vi "CMD_SET_PARAMS.vi"(8 "Max Vel":i32=99, 9 "Chan Ident":string="1", 10 "Accel":i32) -> (0 "ReqCmd":string, 1 "ParamsCmd":string)   [LabVIEW 2017]
panel:
  out "连接的字符串":string
  out "MinVelocity":string
  out "MaxVel":string
  out "Accel":string
  # "（Max Speed/mm）"
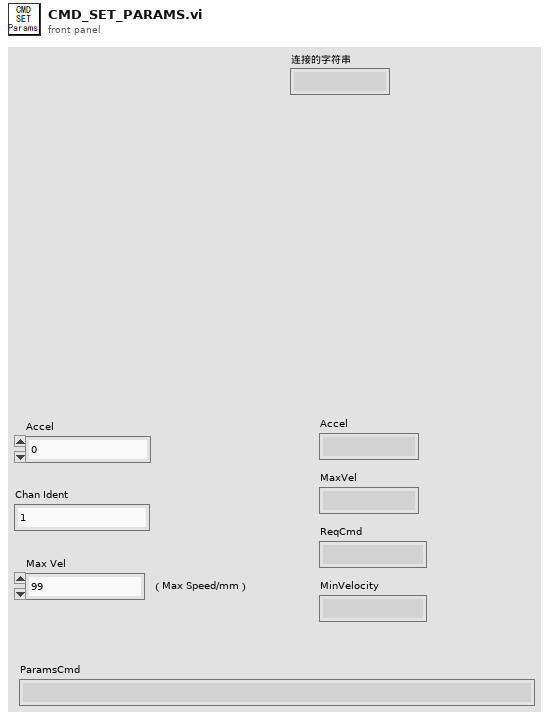
[diagram p1: front panel]
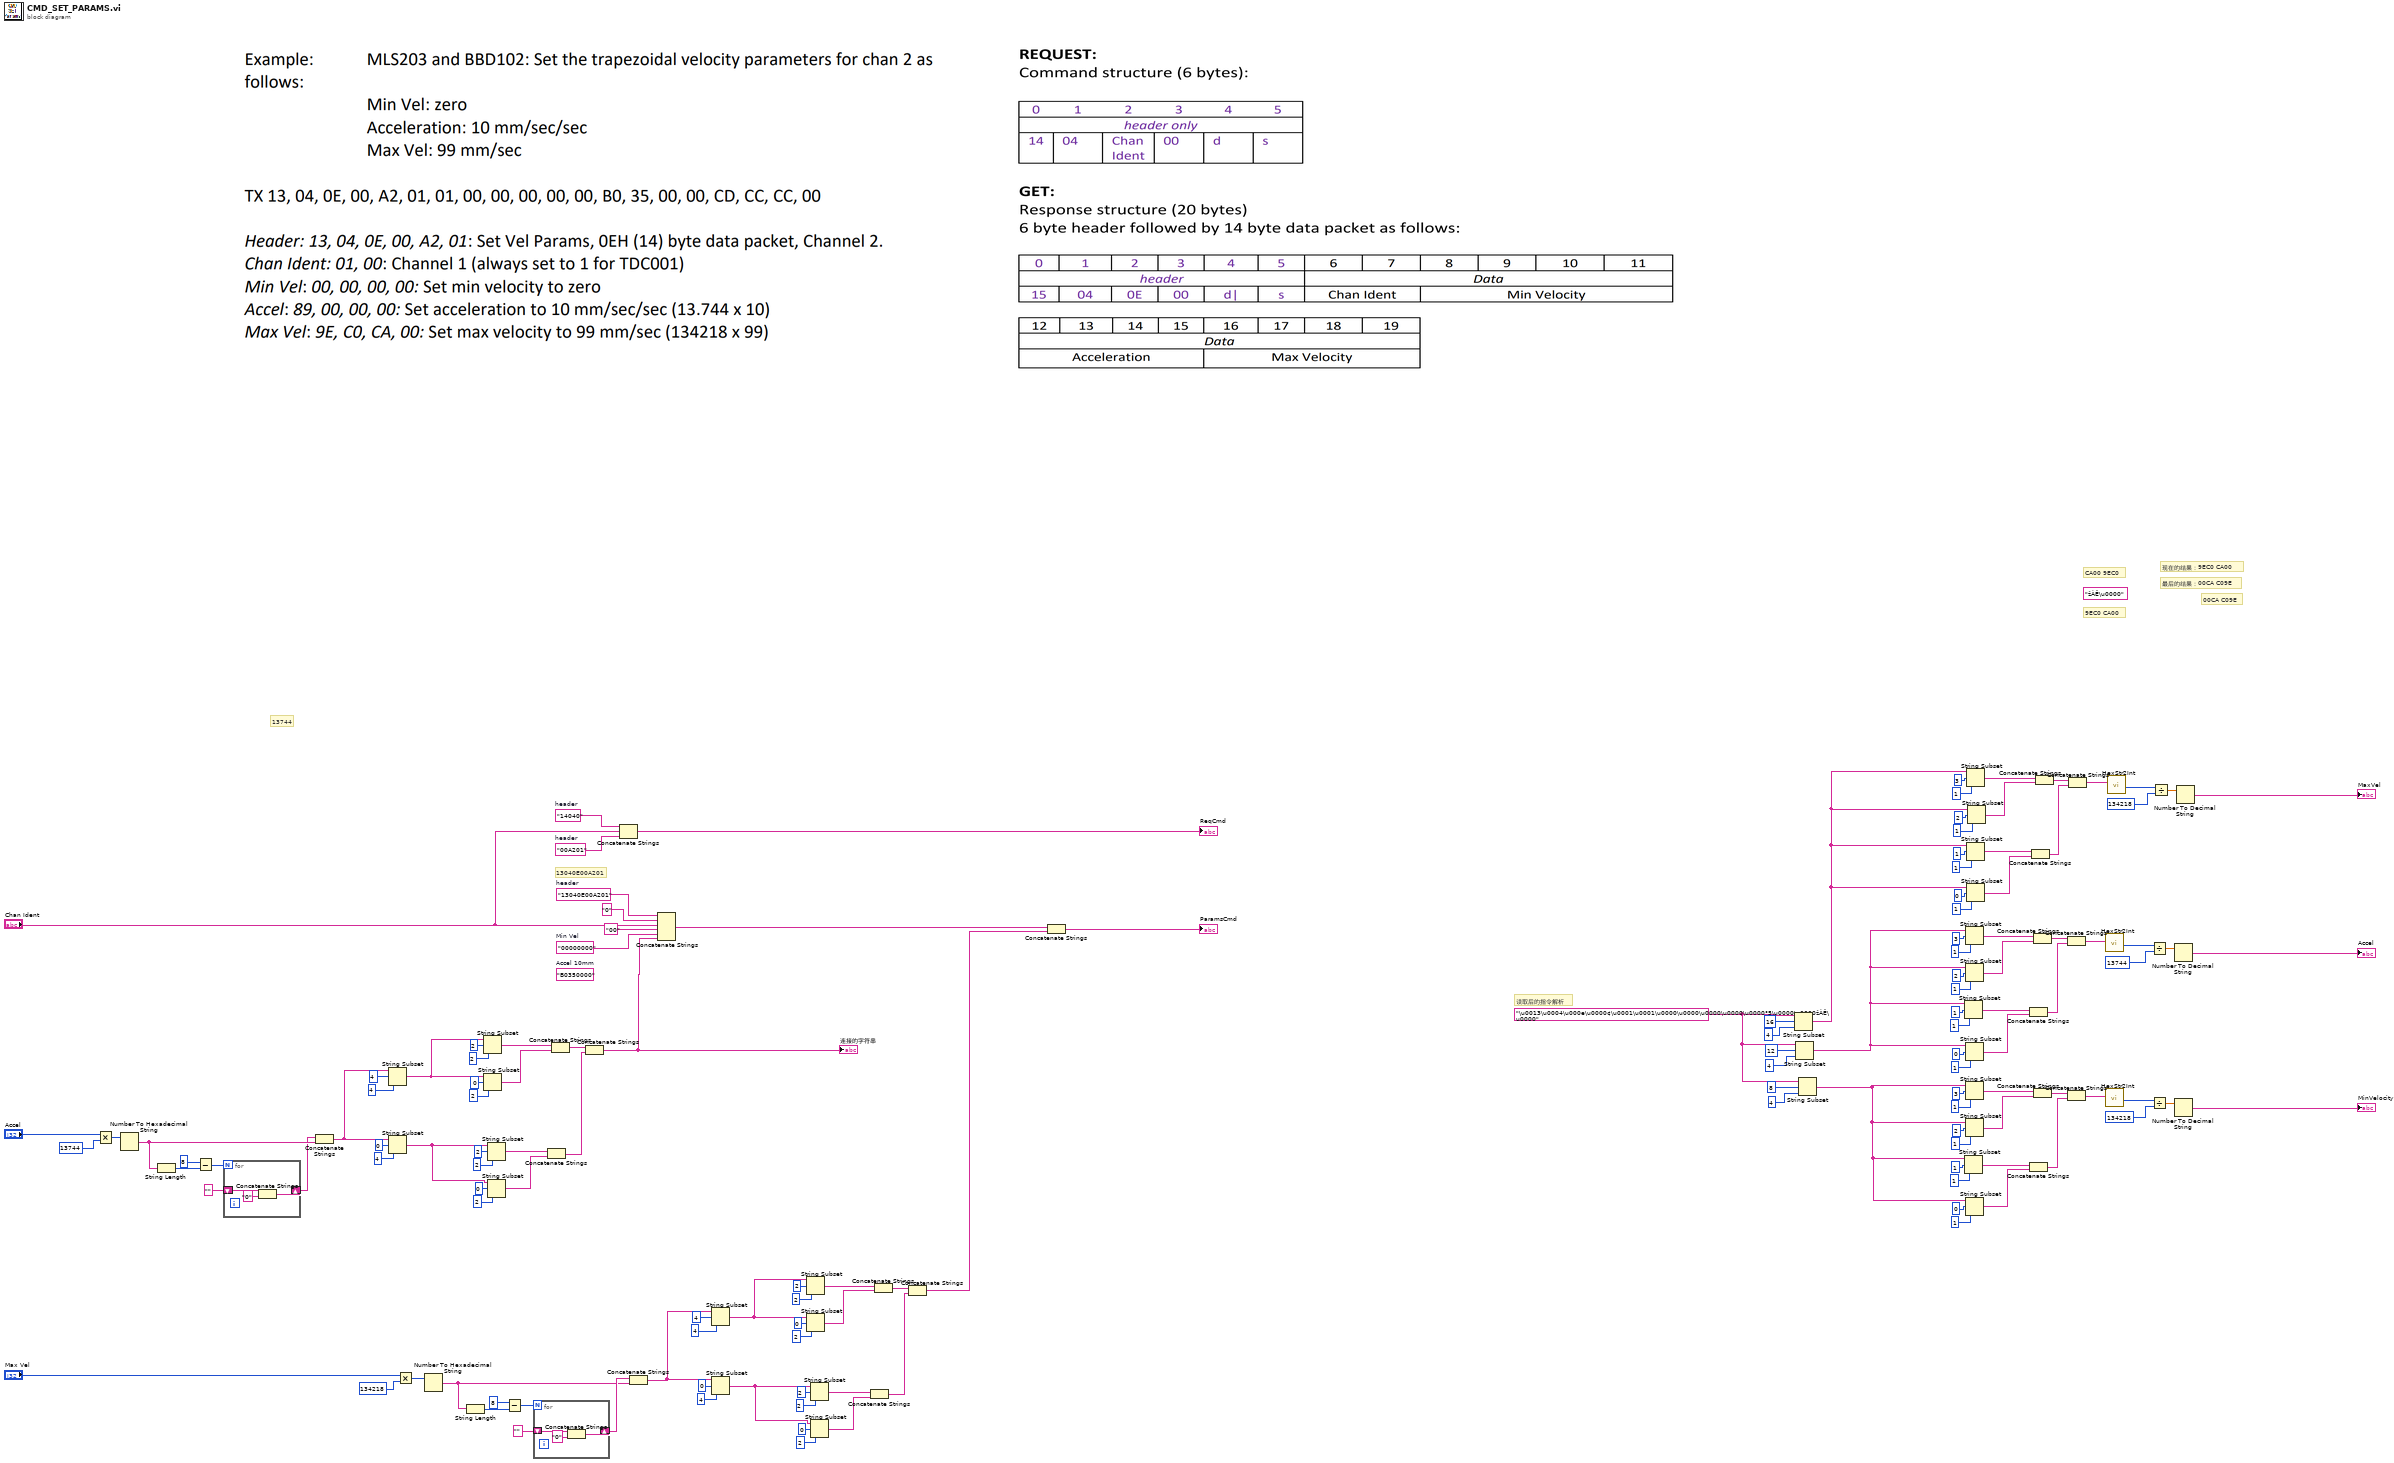
[diagram p0: block diagram]
diagram:
  (unwired) "žÀÊ\u0000" ("MaxVelocity 2")
  w92 = "\u0013\u0004\u000e\u0000¢\u0001\u0001\u0000\u0000\u0000\u0000\u0000°5\u0000\u0000žÀÊ\u0000" ("Hex Display")
  w101 = "00A201"  # header
  w103 = "14040"  # header
  (unwired) "B0350000"  # Accel 10mm
  w108 = "00000000"  # Min Vel
  w110 = "13040E00A201"  # header
  # "13744"
  # "00CA C09E"
  # "现在的结果：9EC0 CA00"
  # "9EC0 CA00"
  # "CA00 9EC0"
  # "最后的结果：00CA C09E"
  # "读取后的指令解析"
  # "13040E00A201"
  n1 = Multiply(x="Accel", y=13744) -> (x*y=w30:i32)
  n2 = Number To Hexadecimal String(2:w30) -> (0:w31:string)  [unwired: 1 in]
  n3 = String Length(string=w31) -> (length=w4:i32)
  n4 = Subtract(x=8, y=w4) -> (x-y=w5:i32)
  n5 = for {
    N: w5 -> [_]
    shift-right: [w140] -> w7
    shift-left: "" -> [w142]
    n6 = Concatenate Strings(w142, "0" ("字符串")) -> (w140:string)
  }
  n7 = Concatenate Strings(w7, w31) -> (w12:string)
  n8 = String Subset(string=w12, offset (0)=4 ("偏移量(0)"), length (rest)=4 ("长度（剩余）")) -> (substring=w17:string)
  n9 = String Subset(string=w12, offset (0)=0 ("偏移量(0)"), length (rest)=4 ("长度（剩余）")) -> (substring=w24:string)
  n10 = Multiply(x="Max Vel", y=134218) -> (x*y=w105:i32)
  n11 = Number To Hexadecimal String(2:w105) -> (0:w104:string)  [unwired: 1 in]
  n12 = String Length(string=w104) -> (length=w138:i32)
  n13 = String Subset(string=w17, offset (0)=2 ("偏移量(0)"), length (rest)=2 ("长度（剩余）")) -> (substring=w18:string)
  n14 = String Subset(string=w17, offset (0)=0 ("偏移量(0)"), length (rest)=2 ("长度（剩余）")) -> (substring=w19:string)
  n15 = String Subset(string=w24, offset (0)=2 ("偏移量(0)"), length (rest)=2 ("长度（剩余）")) -> (substring=w25:string)
  n16 = String Subset(string=w24, offset (0)=0 ("偏移量(0)"), length (rest)=2 ("长度（剩余）")) -> (substring=w26:string)
  n17 = Subtract(x=8, y=w138) -> (x-y=w137:i32)
  n18 = for {
    N: w137 -> [_]
    shift-right: [w143] -> w135
    shift-left: "" -> [w145]
    n19 = Concatenate Strings(w145, "0" ("字符串")) -> (w143:string)
  }
  n20 = Concatenate Strings(w25, w26) -> (w28:string)
  n21 = Concatenate Strings(w18, w19) -> (w27:string)
  n22 = Concatenate Strings(w27, w28) -> (w1:string)
  "连接的字符串" <- w1
  n23 = Concatenate Strings(w103, "Chan Ident", w101) -> (→"ReqCmd":string)
  n24 = Concatenate Strings(w135, w104) -> (w130:string)
  n25 = Concatenate Strings(w110, "0" ("字符串"), "Chan Ident", "00" ("字符串"), w108, w1) -> (w109:string)
  n26 = String Subset(string=w130, offset (0)=4 ("偏移量(0)"), length (rest)=4 ("长度（剩余）")) -> (substring=w125:string)
  n27 = String Subset(string=w130, offset (0)=0 ("偏移量(0)"), length (rest)=4 ("长度（剩余）")) -> (substring=w118:string)
  n28 = String Subset(string=w125, offset (0)=2 ("偏移量(0)"), length (rest)=2 ("长度（剩余）")) -> (substring=w124:string)
  n29 = String Subset(string=w125, offset (0)=0 ("偏移量(0)"), length (rest)=2 ("长度（剩余）")) -> (substring=w123:string)
  n30 = String Subset(string=w118, offset (0)=2 ("偏移量(0)"), length (rest)=2 ("长度（剩余）")) -> (substring=w117:string)
  n31 = String Subset(string=w118, offset (0)=0 ("偏移量(0)"), length (rest)=2 ("长度（剩余）")) -> (substring=w116:string)
  n32 = Concatenate Strings(w117, w116) -> (w114:string)
  n33 = Concatenate Strings(w124, w123) -> (w115:string)
  n34 = Concatenate Strings(w115, w114) -> (w113:string)
  n35 = Concatenate Strings(w109, w113) -> (→"ParamsCmd":string)
  n36 = String Subset(string=w92, offset (0)=16 ("偏移量(0)"), length (rest)=4 ("长度（剩余）")) -> (substring=w74:string)
  n37 = String Subset(string=w92, offset (0)=12 ("偏移量(0)"), length (rest)=4 ("长度（剩余）")) -> (substring=w53:string)
  n38 = String Subset(string=w92, offset (0)=8 ("偏移量(0)"), length (rest)=4 ("长度（剩余）")) -> (substring=w32:string)
  n39 = String Subset(string=w53, offset (0)=1 ("偏移量(0)"), length (rest)=1 ("长度（剩余）")) -> (substring=w64:string)
  n40 = String Subset(string=w32, offset (0)=1 ("偏移量(0)"), length (rest)=1 ("长度（剩余）")) -> (substring=w43:string)
  n41 = String Subset(string=w53, offset (0)=3 ("偏移量(0)"), length (rest)=1 ("长度（剩余）")) -> (substring=w58:string)
  n42 = String Subset(string=w53, offset (0)=0 ("偏移量(0)"), length (rest)=1 ("长度（剩余）")) -> (substring=w65:string)
  n43 = String Subset(string=w32, offset (0)=3 ("偏移量(0)"), length (rest)=1 ("长度（剩余）")) -> (substring=w37:string)
  n44 = String Subset(string=w32, offset (0)=0 ("偏移量(0)"), length (rest)=1 ("长度（剩余）")) -> (substring=w44:string)
  n45 = String Subset(string=w53, offset (0)=2 ("偏移量(0)"), length (rest)=1 ("长度（剩余）")) -> (substring=w59:string)
  n46 = String Subset(string=w32, offset (0)=2 ("偏移量(0)"), length (rest)=1 ("长度（剩余）")) -> (substring=w38:string)
  n47 = String Subset(string=w74, offset (0)=1 ("偏移量(0)"), length (rest)=1 ("长度（剩余）")) -> (substring=w81:string)
  n48 = String Subset(string=w74, offset (0)=3 ("偏移量(0)"), length (rest)=1 ("长度（剩余）")) -> (substring=w87:string)
  n49 = String Subset(string=w74, offset (0)=0 ("偏移量(0)"), length (rest)=1 ("长度（剩余）")) -> (substring=w80:string)
  n50 = String Subset(string=w74, offset (0)=2 ("偏移量(0)"), length (rest)=1 ("长度（剩余）")) -> (substring=w86:string)
  n51 = Concatenate Strings(w64, w65) -> (w67:string)
  n52 = Concatenate Strings(w43, w44) -> (w46:string)
  n53 = Concatenate Strings(w81, w80) -> (w78:string)
  n54 = Concatenate Strings(w58, w59) -> (w66:string)
  n55 = Concatenate Strings(w37, w38) -> (w45:string)
  n56 = Concatenate Strings(w87, w86) -> (w79:string)
  n57 = Concatenate Strings(w66, w67) -> (w68:string)
  n58 = Concatenate Strings(w45, w46) -> (w47:string)
  n59 = Concatenate Strings(w79, w78) -> (w77:string)
  n60 = call "HexStr2Int.vi"("十六进制字符串"=w68) -> ("数字"=w69:u32)  [unwired: 10 in]
  n61 = call "HexStr2Int.vi"("十六进制字符串"=w47) -> ("数字"=w48:u32)  [unwired: 10 in]
  n62 = call "HexStr2Int.vi"("十六进制字符串"=w77) -> ("数字"=w76:u32)  [unwired: 10 in]
  n63 = Divide(x=w69, y=13744) -> (x/y=w71:dbl)
  n64 = Divide(x=w48, y=u32 134218) -> (x/y=w50:dbl)
  n65 = Divide(x=w76, y=u32 134218) -> (x/y=w73:dbl)
  n66 = Number To Decimal String(number=w71) -> (decimal integer string=→"Accel":string)  [unwired: 1 in]
  n67 = Number To Decimal String(number=w50) -> (decimal integer string=→"MinVelocity":string)  [unwired: 1 in]
  n68 = Number To Decimal String(number=w73) -> (decimal integer string=→"MaxVel":string)  [unwired: 1 in]
